vi "BordersPercents2BordersPixels.vi"(10 "Borders in":T2, 11 "Bounds":T1) -> (3 "Borders out":T2)   [LabVIEW 2022 SP3, in "PentaPanesLibrary.lvlib" / "PentaPanes.lvclass"]
doc: "This VI converts Borders with percent units to pixels units using Bounds Width and Height values as a 100%."
uses:
  PentaPanes.lvclass
  BordersCluster.ctl
  <vilib>/Utility/miscctls.llb/LVBoundsTypeDef.ctl
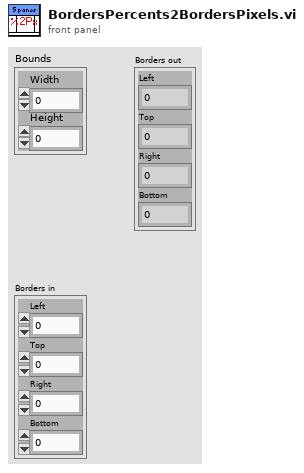
[diagram p1: front panel]
types:
  T1 = typedef "LVBoundsTypeDef.ctl" = cluster{"Width":i32, "Height":i32}
  T2 = typedef "PentaPanesLibrary.lvlib/PentaPanes.lvclass/BordersCluster.ctl" = cluster{"Left":i32, "Top":i32, "Right":i32, "Bottom":i32}
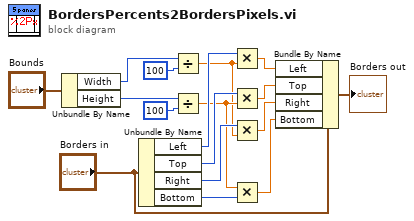
[diagram p0: block diagram]
diagram:
  n1 = Unbundle By Name("Bounds") -> ("Width"=w2:i32, "Height"=w3:i32)
  n2 = Unbundle By Name("Borders in") -> ("Left"=w8:i32, "Top"=w9:i32, "Right"=w10:i32, "Bottom"=w11:i32)
  n3 = Divide(x=w2, y=u32 100) -> (x/y=w6:dbl)
  n4 = Divide(x=w3, y=u32 100) -> (x/y=w7:dbl)
  n5 = Multiply(x=w8, y=w6) -> (x*y=w12:dbl)
  n6 = Multiply(x=w9, y=w7) -> (x*y=w13:dbl)
  n7 = Multiply(x=w10, y=w6) -> (x*y=w14:dbl)
  n8 = Multiply(x=w7, y=w11) -> (x*y=w15:dbl)
  n9 = Bundle By Name(cluster="Borders in", "Left"=w12, "Top"=w13, "Right"=w14, "Bottom"=w15) -> (→"Borders out":T2)
